vi "Verify Path.vi"(8 "error in":errorcluster, 11 "Launcher in":refnum<class "Launcher.lvclass">) -> (0 "error out":errorcluster, 2 "Abort?":bool, 3 "Launcher out":refnum<class "Launcher.lvclass">)   [LabVIEW 2019, in "Launcher.lvlib" / "Launcher.lvclass"]
uses:
  Library/Launcher.lvclass
  Library/Launcher.lvclass/Launcher.ctl
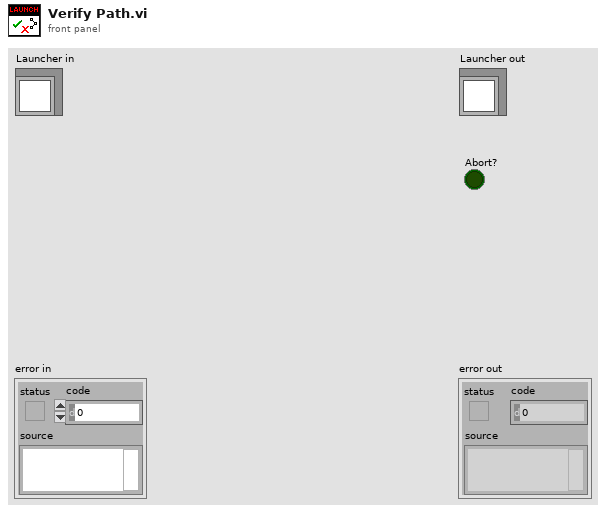
[diagram p1: front panel]
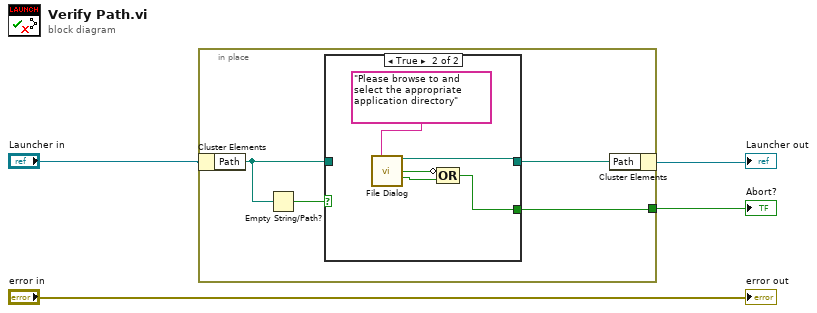
[diagram p0: block diagram]
diagram:
  n1 = in-place {
    in-place-border: [w5] -> w1
    n2 = in-place-cluster #1("Launcher in") -> ("Path"=w7:path)
    n3 = Empty String/Path?(string/path=w7) -> (empty?=w8:bool)
    n4 = case shown="True" w8 {
      tunnel: w7 -> [w9 _]
      tunnel: [w9 w13] -> w6
      tunnel: [_ w10] -> w5
      frame False {
      }
      frame True {
        n5 = call "File Dialog"("prompt"="Please browse to and select the appropriate application directory") -> ("selected path"=w13:path, "exists"=w12:bool, "cancelled"=w11:bool)  [unwired: 11 in, 1 out]
        n6 = Compound Arithmetic op=OR(invert w12, w11) -> (w10:bool)
      }
    }
    n7 = in-place-cluster #1("Path"=w6) -> (→"Launcher out":refnum<class "Launcher.lvclass">)
  }
  "Abort?" <- w1
  "error out" <- "error in"
